vi "worksheet write datetime.vi"(6 "format":u32, 7 "datetime":T1, 8 "error in (no error)":errorcluster, 9 "col":u16, 10 "row":u32, 11 "worksheet":u32) -> (0 "error out":errorcluster, 3 "function return":u32(ring), 5 "datetime out":T1)   [LabVIEW 2015, in "xlsxwriter.lvlib"]
doc: "lxw_error worksheet_write_datetime(lxw_worksheet worksheet, lxw_row_t row, lxw_col_t col, lxw_datetime *datetime, lxw_format format);"
uses:
  xlsxwriter.lvlib
  xlsxwriter.dll
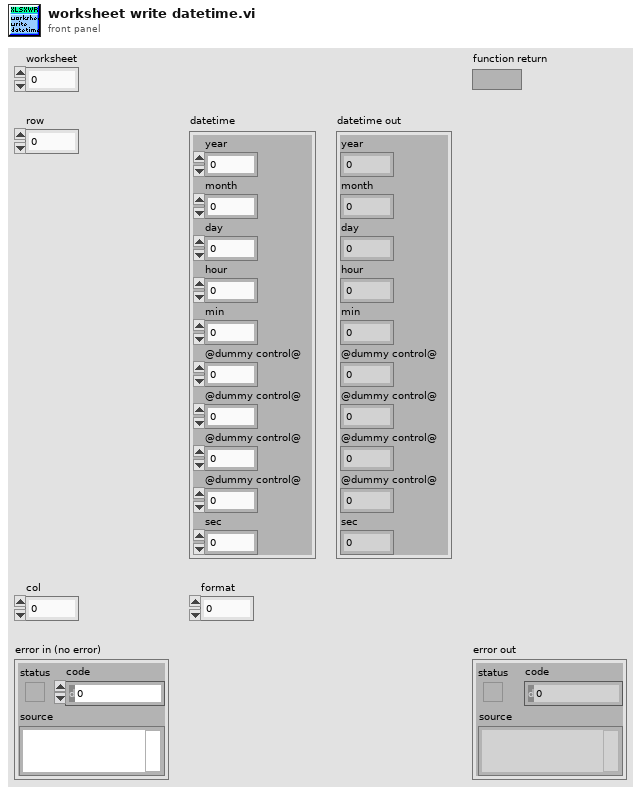
[diagram p1: front panel]
types:
  T1 = cluster{"year":i32, "month":i32, "day":i32, "hour":i32, "min":i32, "@dummy control@":i8, "@dummy control@":i8, "@dummy control@":i8, "@dummy control@":i8, "sec":dbl}
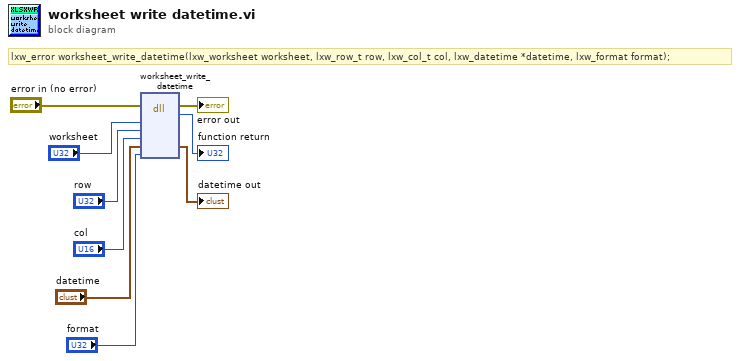
[diagram p0: block diagram]
diagram:
  # "lxw_error worksheet_write_datetime(lxw_worksheet worksheet, lxw_row_t row, lxw_col_t col, lxw_datetime *datetime, lxw_format format);"
  n1 = dll-call lib="C:/Users/WDAGUtilityAccount/Desktop/lv_vis_added_cell/xlsxwriter.*" fn="worksheet_write_datetime"(error in="error in (no error)", "worksheet"="worksheet", "row"="row", "col"="col", "datetime"="datetime", "format"="format") -> (error out=→"error out":errorcluster, →"function return":u32, "datetime"=→"datetime out":T1)  [unwired: 6 in, 1 out]
